vi "MACBIN Read Header__ogtk.vi"(6 "error in (no error)":errorcluster, 7 "resource file":path, 8 "data file":path, 9 "macbinary file":path) -> (0 "error out":errorcluster, 1 "res file refnum":refnum<file>, 2 "data filerefnum":refnum<file>, 3 "macbin filerefnum":refnum<file>, 4 "data length":i32, 5 "res length":i32)   [LabVIEW 2016]
uses:
  <userlib>/_OpenG.lib/lvzip/macbin.llb/MACBIN Resource Header__ogtk.ctl
panel:
  in  "finder info":T1 {"mod date" format="%<%H:%M:%S\n%m/%d/%Y>T"; "creation date" format="%<%H:%M:%S\n%m/%d/%Y>T"}
  # "Please visit http://www.OpenG.org to learn about the\nOpen Source LabVIEW software movement.\n\nNOTICE -- YOU MUST LEAVE THIS NOTICE IN PLACE.  PER THE TERMS OF THE LICENSE BELOW, YOU MAY SUBLICENSE THIS SOFTWARE \nIN ANY WAY THAT DOES NOT CONFLICT WITH THIS LICENSE.\n\n### BSD License (http://www.opensource.org/licenses/bsd-license.php) Begin ###\n \nCopyright (C) 2002 Christophe Salzmann christophe.salzmann@epfl.ch\nCopyright (C) 2002 Rolf Kalbermatter rolf.kalbermatter@citengineering.com\n\nAll rights reserved.\n\nRedistribution and use in source and binary forms, with or without modification, are permitted provided that the following conditions are met:\n\n    * Redistributions of source code must retain the above copyright notice, this list of conditions and the following disclaimer.\n    * Redistributions in binary form must reproduce the above copyright notice, this list of conditions and the following disclaimer in the \n       documentation and/or other materials provided with the distribution.\n    * Neither the name of SciWare, James Kring, Inc., nor the names of its contributors may be used to endorse or promote products derived \n       from this software without specific prior written permission.\n\nTHIS SOFTWARE IS PROVIDED BY THE COPYRIGHT HOLDERS AND CONTRIBUTORS \"AS IS\" AND ANY EXPRESS OR IMPLIED WARRANTIES, \nINCLUDING, BUT NOT LIMITED TO, THE IMPLIED WARRANTIES OF MERCHANTABILITY AND FITNESS FOR A PARTICULAR PURPOSE ARE \nDISCLAIMED. IN NO EVENT SHALL THE COPYRIGHT OWNER OR CONTRIBUTORS BE LIABLE FOR ANY DIRECT, INDIRECT, INCIDENTAL,\n SPECIAL, EXEMPLARY, OR CONSEQUENTIAL DAMAGES (INCLUDING, BUT NOT LIMITED TO, PROCUREMENT OF SUBSTITUTE GOODS OR \nSERVICES; LOSS OF USE, DATA, OR PROFITS; OR BUSINESS INTERRUPTION) HOWEVER CAUSED AND ON ANY THEORY OF LIABILITY, \nWHETHER IN CONTRACT, STRICT LIABILITY, OR TORT (INCLUDING NEGLIGENCE OR OTHERWISE) ARISING IN ANY WAY OUT OF THE USE \nOF THIS SOFTWARE, EVEN IF ADVISED OF THE POSSIBILITY OF SUCH DAMAGE.\n\n### BSD License End ###"
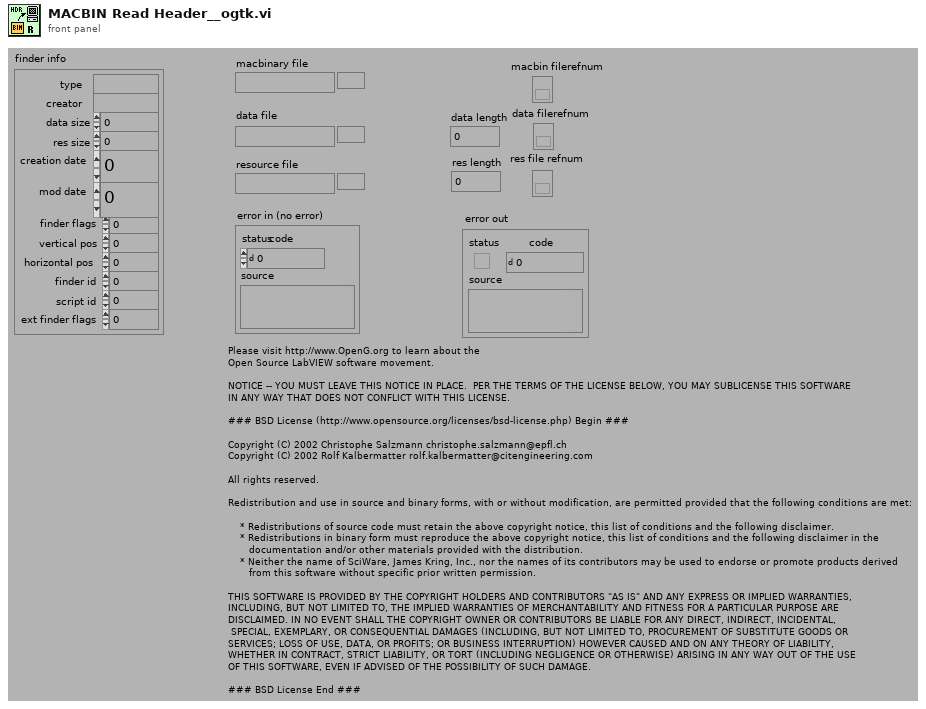
[diagram p1: front panel]
types:
  T1 = typedef "MACBIN Resource Header__ogtk.ctl" = cluster{"type":string, "creator":string, "data size":u32, "res size":u32, "creation date":u32, "mod date":u32, "finder flags":u16, "vertical pos":i16, "horizontal pos":i16, "finder id":u16, "script id":u8, "ext finder flags":u8}
  T2 = typedef "MACBIN Macbinary Header__ogtk.ctl" = cluster{"Finder flags":u8, "zero0":u8, "vertical pos":u16, "horizontal pos":u16, "finder id":u16, "protected":u8, "zero1":u8, "data length":i32, "res length":i32, "creation date":u32, "last mod":u32, "comment length":i16, "Finder flags 2":u8, "file identifier":u32, "script id":u8, "ext finder flags":u8, "zero2":i32, "zero3":i32, "total length":u32, "sec hdr length":u16, "creator version":u8, "minimum version":u8}
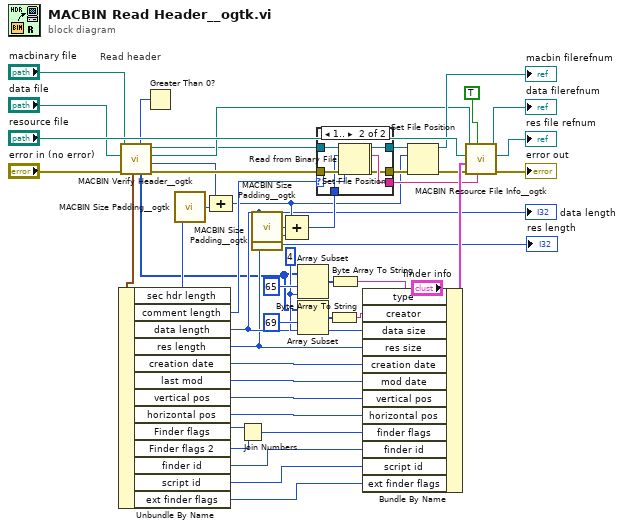
[diagram p0: block diagram]
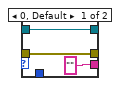
[diagram p2: hidden frame]
diagram:
  w40 = 4
  # "Read header"
  n1 = call <userlib>:"MACBIN Verify Header__ogtk.vi"("error in (no error)"="error in (no error)", "macbinary file"="data file", "data file"="macbinary file") -> ("error out"=w6:errorcluster, "file offset"=w3:i32, "data file out"=w8:path, "file refnum"=w1:refnum<file>, "header bytes"=w7:u8[], "macbinary version"=w9:i32, "macbinary header"=w10:T2)  [unwired: 2 in]
  n2 = Unbundle By Name(w10) -> ("sec hdr length"=w16:u16, "comment length"=w22:i16, "data length"=w12:i32, "res length"=w11:i32, "creation date"=w36:u32, "last mod"=w31:u32, "vertical pos"=w28:u16, "horizontal pos"=w35:u16, "Finder flags"=w27:u8, "Finder flags 2"=w26:u8, "finder id"=w37:u16, "script id"=w38:u8, "ext finder flags"=w39:u8)
  "data length" <- w12
  "res length" <- w11
  n3 = Greater Than 0?(x=w9) -> ()  [unwired: 1 out]
  n4 = call <userlib>:"MACBIN Size Padding__ogtk.vi"("length"=w16) -> ("padded length"=w15:i32)  [unwired: 4 in]
  n5 = Compound Arithmetic op=ADD(w3, w15) -> (w17:i32)
  n6 = Join Numbers(hi=w27, lo=w26) -> ((hi.lo)=w25:u16)
  n7 = call <userlib>:"MACBIN Size Padding__ogtk.vi"("length"=w12) -> ("padded length"=w14:i32)  [unwired: 4 in]
  n8 = call <userlib>:"MACBIN Size Padding__ogtk.vi"("length"=w11) -> ("padded length"=w13:i32)  [unwired: 4 in]
  n9 = Compound Arithmetic op=ADD(w17, w14, w13) -> (w23:i32)
  n10 = Array Subset(array=w7, index=65 ("Array Index"), length=w40) -> (w44:u8[])
  n11 = Array Subset(array=w7, index=69 ("Array Index"), length=w40) -> (w43:u8[])
  n12 = case shown="1.." w22 {
    selector: w22 -> [_ w56]
    tunnel: w6 -> [w51 w60]
    tunnel: w1 -> [w50 w59]
    tunnel: ["" w58] -> w24
    tunnel: [w51 w55] -> w21
    tunnel: [w50 w54] -> w20
    tunnel: w23 -> [_ w57]
    frame 0, Default {
    }
    frame 1.. {
      n13 = Set File Position(offset (in bytes) (0)=w57, refnum=w59, error in=w60) -> (refnum out=w53:refnum<file>, error out=w52:errorcluster)  [unwired: 1 in]
      n14 = Read from Binary File(8:w52, 10:w56, 11:w53) -> (0:w55:errorcluster, 2:w58:string, 3:w54:refnum<file>)  [unwired: 3 in, 1 out]
    }
  }
  n15 = Byte Array To String(unsigned byte array=w43) -> (string=w29:string)
  n16 = Byte Array To String(unsigned byte array=w44) -> (string=w30:string)
  n17 = Bundle By Name(cluster="finder info", "type"=w30, "creator"=w29, "data size"=w12, "res size"=w11, "creation date"=w36, "mod date"=w31, "vertical pos"=w28, "horizontal pos"=w35, "finder flags"=w25, "finder id"=w37, "script id"=w38, "ext finder flags"=w39) -> (w32:T1)
  n18 = Set File Position(offset (in bytes) (0)=w17, refnum=w20, error in=w21) -> (refnum out=→"macbin filerefnum":refnum<file>, error out=w18:errorcluster)  [unwired: 1 in]
  n19 = call <userlib>:"MACBIN Resource File Info__ogtk.vi"("comment"=w24, "write (F)"=TRUE, "error in (no error)"=w18, "file info"=w32, "resource file"="resource file", "data file"=w8) -> ("error out"=→"error out":errorcluster, "resource refnum"=→"res file refnum":refnum<file>, "data refnum"=→"data filerefnum":refnum<file>)  [unwired: 1 in, 2 out]
